vi "Transfer2.vi"   [LabVIEW 2021]
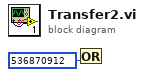
[diagram p0: block diagram]
diagram:
  n1 = Or(y=u32 536870912) -> (x=w1:u32)  [unwired: 1 out]
